vi "Get Firebase Recovery_SN.vi"(8 "error in (no error)":errorcluster caption="entrée d'erreur (pas d'erreur)", 11 "Creation_SN Database (Default) en entrée":refnum<class "Creation_SN Database (Default).lvclass">) -> (0 "error out":errorcluster caption="sortie d'erreur", 2 "Library FireBase.lvlib:Firebase Recovery_SN.lvclass":refnum<class "Firebase Recovery_SN.lvclass">, 3 "Creation_SN Database (Default) en sortie":refnum<class "Creation_SN Database (Default).lvclass">)   [LabVIEW 2020, in "Library Instrument & Equipement.lvlib" / "Library Creation_SN.lvlib" / "Creation_SN Database (Default).lvclass"]
uses:
  Creation_SN Database (Default).lvclass
  Firebase/Source/Firebase Recovery_SN/Firebase Recovery_SN.lvclass
  Creation_SN Database (Default).lvclass/Creation_SN Database (Default).ctl
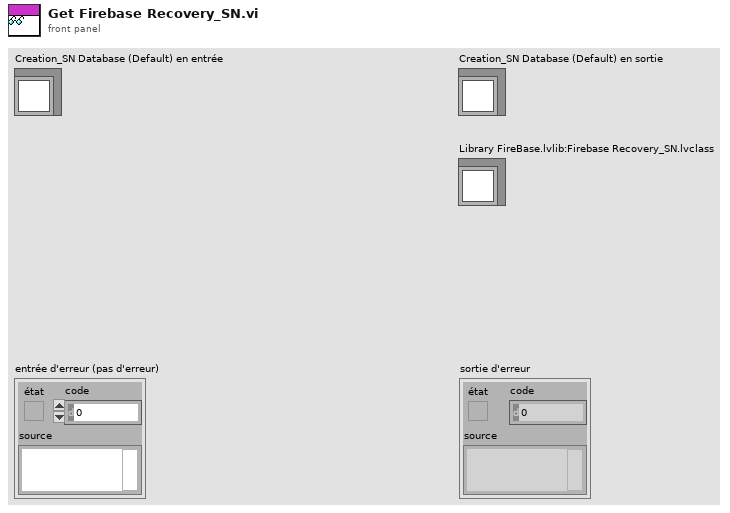
[diagram p1: front panel]
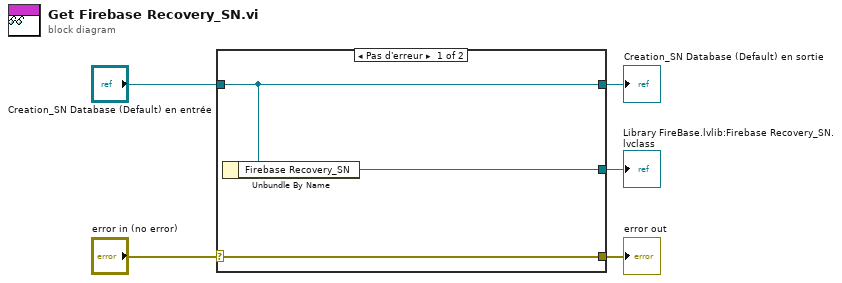
[diagram p0: block diagram]
diagram:
  n1 = case shown="Pas d'erreur" "error in (no error)" {
    selector: "error in (no error)" -> [w8 w9]
    tunnel: [w8 w9] -> w4
    tunnel: [w7 w10] -> w2
    tunnel: "Creation_SN Database (Default) en entrée" -> [w7 w10]
    tunnel: [w6 _] -> w1
    frame No Error {
      n2 = Unbundle By Name(w7) -> ("Firebase Recovery_SN"=w6:refnum<class "Firebase Recovery_SN.lvclass">)
    }
    frame Error {
    }
  }
  "error out" <- w4
  "Creation_SN Database (Default) en sortie" <- w2
  "Library FireBase.lvlib:Firebase Recovery_SN.lvclass" <- w1
